vi "getUpdateAmountStatement.vi"(8 "error in (no error)":errorcluster, 11 "Goal in":refnum<class "Goal.lvclass">) -> (0 "error out":errorcluster, 2 "Update Statement":string, 3 "Goal out":refnum<class "Goal.lvclass">)   [LabVIEW 2018, in "Goal.lvclass"]
uses:
  Goal.lvclass
  Goal.lvclass/Goal.ctl
  Category/Category.lvclass
  WhichMonth/WhichMonth.lvclass
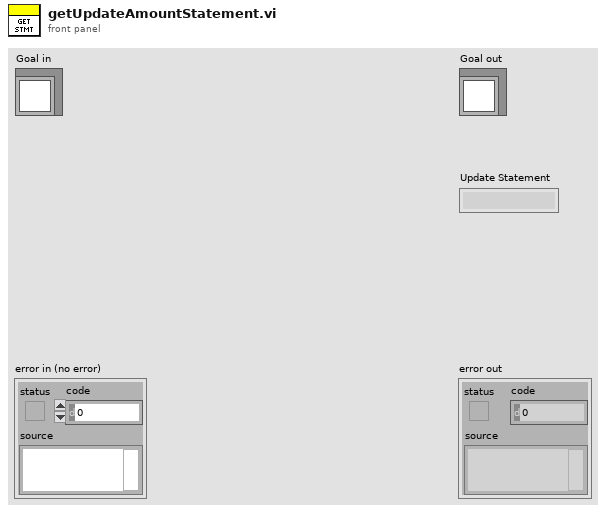
[diagram p1: front panel]
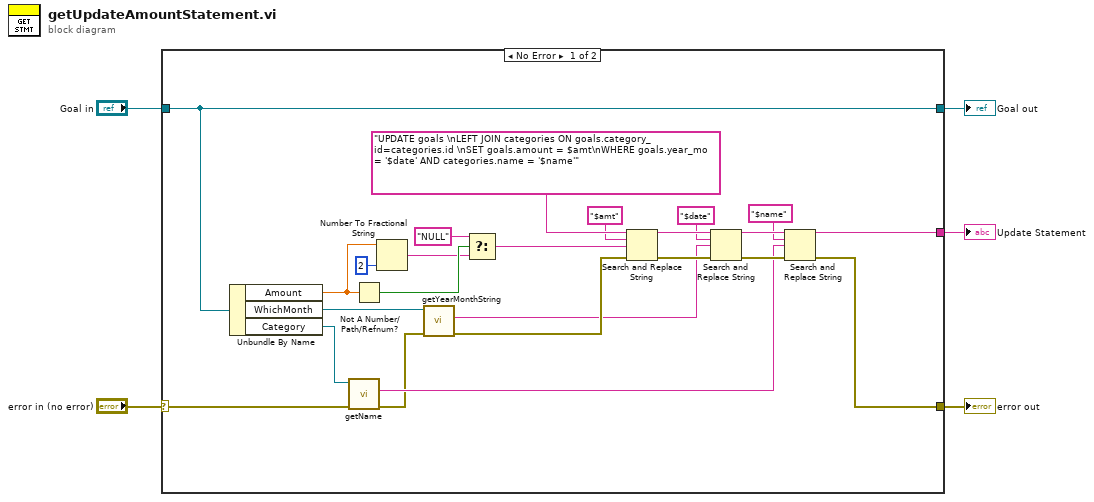
[diagram p0: block diagram]
diagram:
  n1 = case shown="No Error" "error in (no error)" {
    selector: "error in (no error)" -> [w17 w31]
    tunnel: [w20 w31] -> w4
    tunnel: [w23 w30] -> w2
    tunnel: "Goal in" -> [w23 w30]
    tunnel: [w15 _] -> w1
    frame No Error {
      n2 = Unbundle By Name(w23) -> ("Amount"=w14:dbl, "WhichMonth"=w9:refnum<class "WhichMonth.lvclass">, "Category"=w18:refnum<class "Category.lvclass">)
      n3 = call "getName.vi"("error in (no error)"=w17, "Category in"=w18) -> ("error out"=w8:errorcluster, "Name"=w16:string)  [unwired: 7 in, 1 out]
      n4 = Not A Number/Path/Refnum?(number/path/refnum=w14) -> (NaN/Path/Refnum?=w13:bool)
      n5 = Number To Fractional String(number=w14, precision (6)=i16 2) -> (F-format string=w12:string)  [unwired: 2 in]
      n6 = call "getYearMonthString.vi"("error in (no error)"=w8, "WhichMonth in"=w9) -> ("error out"=w7:errorcluster, "Year-Month"=w6:string)  [unwired: 7 in, 1 out]
      n7 = Select(t="NULL", s=w13, f=w12) -> (s? t:f=w10:string)
      n8 = Search and Replace String(input string="UPDATE goals \nLEFT JOIN categories ON goals.category_id=categories.id \nSET goals.amount = $amt\nWHERE goals.year_mo = '$date' AND categories.name = '$name'", search string="$amt", replace string=w10, error in=w7) -> (result string=w27:string, error out=w29:errorcluster)  [unwired: 4 in, 2 out]
      n9 = Search and Replace String(input string=w27, search string="$date", replace string=w6, error in=w29) -> (result string=w21:string, error out=w22:errorcluster)  [unwired: 4 in, 2 out]
      n10 = Search and Replace String(input string=w21, search string="$name", replace string=w16, error in=w22) -> (result string=w15:string, error out=w20:errorcluster)  [unwired: 4 in, 2 out]
    }
    frame Error {
    }
  }
  "error out" <- w4
  "Goal out" <- w2
  "Update Statement" <- w1
